vi "连接字符串.vi"(1 "Separator (,)":string="," caption="分隔符(,)", 2 "Strings In":string[](array[string]) caption="字符串输入") -> (0 "String":string caption="字符串")   [LabVIEW 2012]
doc: "Joins the elements of <B>Strings In</B> separating them with <B>Separator</B>.\n\n<B>Separator</B> - The item to put between each string.\n<B>Strings In</B> - The strings to join.\n<B>String</B> - The resultant joined string."
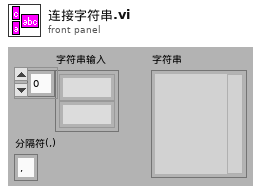
[diagram p1: front panel]
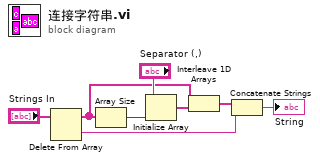
[diagram p0: block diagram]
diagram:
  n1 = Delete From Array(array="Strings In") -> (deleted portion=w2:string, array with subset deleted=w5:string[])  [unwired: 2 in]
  n2 = Array Size(array=w5) -> (size(s)=w6:i32)
  n3 = Initialize Array("Separator (,)", w6) -> (w4:string[])
  n4 = Interleave 1D Arrays(w5, w4) -> (w3:string[])
  n5 = Concatenate Strings(w3, w2) -> (→"String":string)
